vi "9174_9227_9205_CV_test.vi"() -> ()   [LabVIEW 2018]
uses:
  <vilib>/Utility/sysdir.llb/System Directory Type.ctl
panel:
  in  "觸發顯示訊號":bool=TRUE
  out "DW 2":bool
  out "ON":bool
  in  "自動存檔開關":bool=TRUE
  out "DW":bool
  in  "Stop":bool
  out "Time":timestamp format="%<%x %.3X>T"
  out "Real-Time":dynamicdata(graph)
  out "Real-Time":dynamicdata(graph)
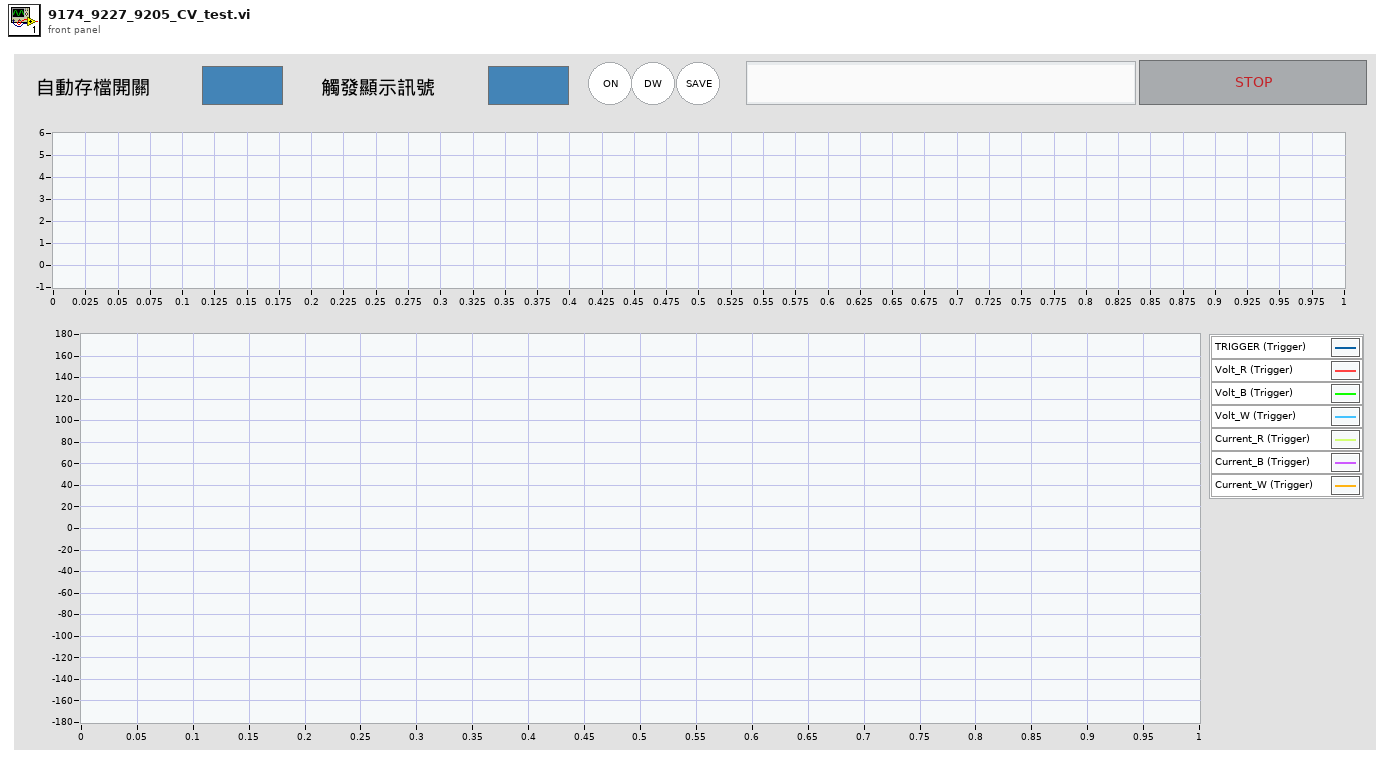
[diagram p1: front panel]
types:
  T1 = typedef "System Directory Type.ctl" = i32
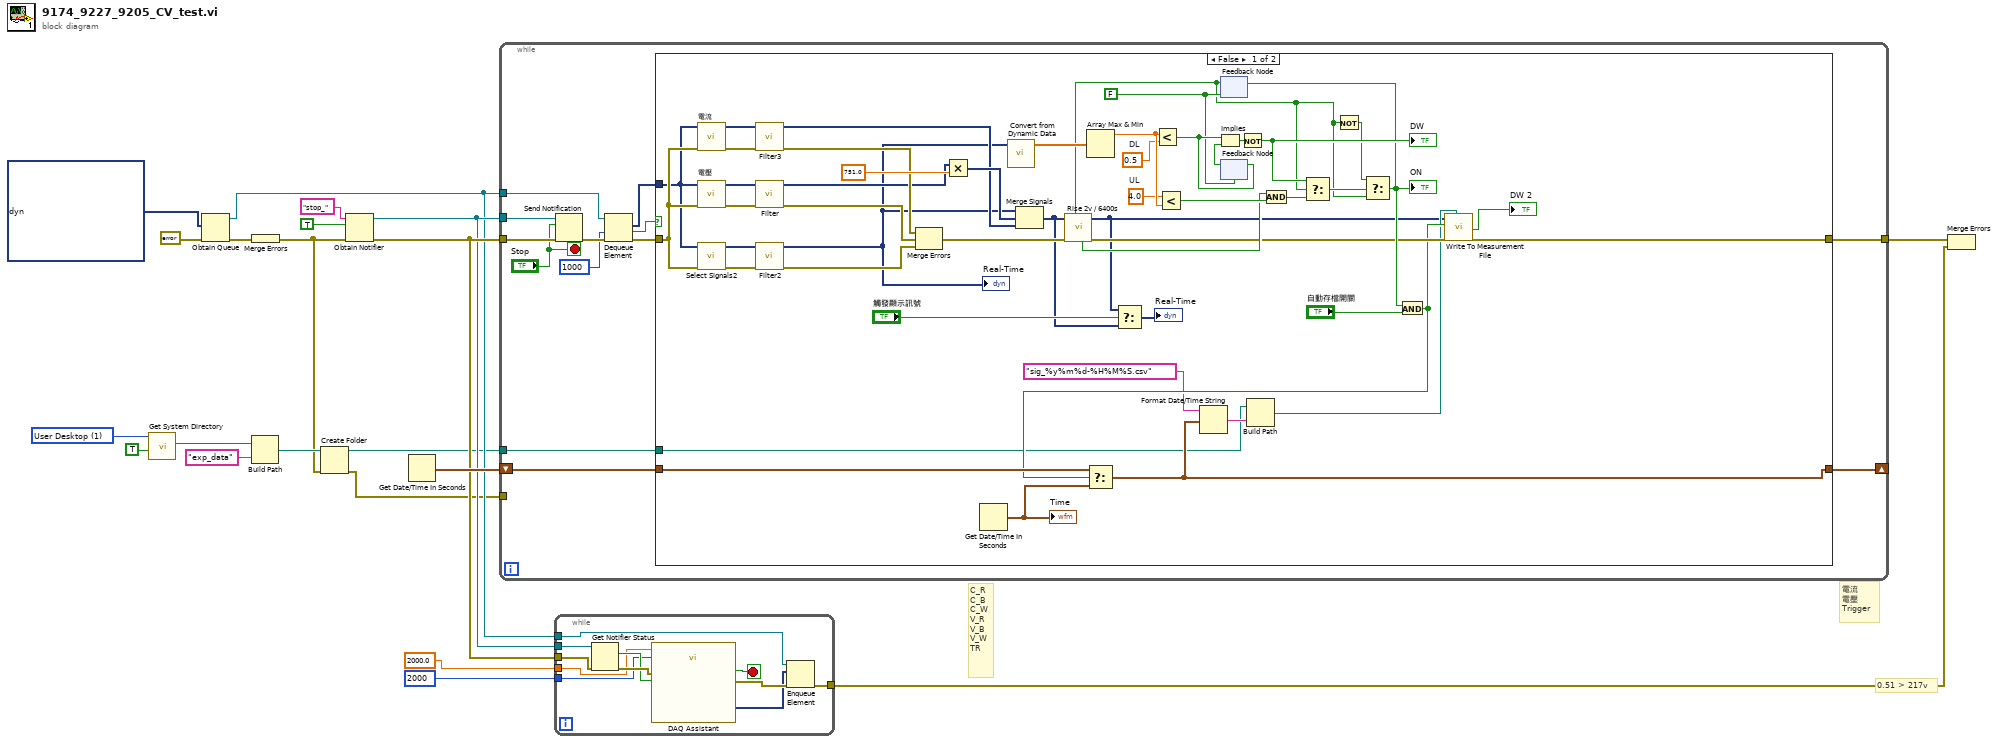
[diagram p0: block diagram]
diagram:
  w5 = T1 1 items=["User Home"=0, "User Desktop"=1, "User Documents"=2, "User Application Data"=3, "User Preferences"=4, "User Temporary"=5, "Public Documents"=6, "Public Application Data"=7, "Public Preferences"=8, "Public Cache"=13, "System Core Libraries"=9, "System Installed Libraries"=10, "Application Files"=11, "Boot Volume Root"=12] ("system directory type")
  # "C_R\nC_B\nC_W\nV_R\nV_B\nV_W\nTR"
  # "0.51 > 217v"
  # "電流\n電壓\nTrigger"
  n1 = call <vilib>:"Get System Directory.vi"("create directory if not found? (F)"=TRUE, "system directory type"=w5) -> ("system directory"=w7:path)  [unwired: 9 in]
  n2 = Obtain Queue(element data type=dynamicdata [] ("data"), error in (no error)=errorcluster {"status"=FALSE, "code"=0, "source"=""} ("Error In")) -> (queue out=w9:refnum<queue>, error out=w21:errorcluster)  [unwired: 3 in, 1 out]
  n3 = Build Path(base path=w7, name or relative path="exp_data") -> (appended path=w4:path)
  n4 = Merge Errors(w21) -> (w1:errorcluster)
  n5 = Create Folder(path (use dialog)=w4, error in=w1) -> (created path=w3:path, error out=w2:errorcluster)  [unwired: 1 in, 1 out]
  n6 = Obtain Notifier(name (unnamed)="stop_", notification data type=TRUE, error in (no error)=w1) -> (notifier out=w15:refnum<notifier>, error out=w16:errorcluster)  [unwired: 1 in, 1 out]
  n7 = Get Date/Time In Seconds() -> (seconds since 1Jan1904=w17:timestamp)
  n8 = while {
    tunnel: w16 -> [w34]
    tunnel: w15 -> [w33]
    tunnel: [w26] -> w10
    shift-right: [w31] -> _
    shift-left: w17 -> [w32]
    tunnel: w9 -> [w29]
    tunnel: w3 -> [w23]
    tunnel: w2 -> [_]
    stop <- "Stop" stop-if-true
    n9 = Send Notification(notification="Stop", notifier=w33, error in (no error)=w34) -> (error out=w30:errorcluster)  [unwired: 1 out]
    n10 = Dequeue Element(queue=w29, timeout in ms (-1)=1000, error in (no error)=w30) -> (element=w22:dynamicdata, timed out?=w27:bool, error out=w25:errorcluster)  [unwired: 1 out]
    n11 = case shown="False" w27 {
      tunnel: w32 -> [w83 w85]
      tunnel: [w42 w85] -> w31
      tunnel: w22 -> [w78 _]
      tunnel: [w68 w84] -> w26
      tunnel: w25 -> [w79 w84]
      tunnel: w23 -> [w40 _]
      frame False {
        w53 = FALSE
        w52 = 4.0  # UL
        w51 = 0.5  # DL
        n12 = call "電流"("error in (no error)"=w79, "Signals"=w78) -> ("error out"=w74:errorcluster, "Signal Out"=w76:dynamicdata)  [unwired: 8 in]
        n13 = call "電壓"("error in (no error)"=w79, "Signals"=w78) -> ("error out"=w80:errorcluster, "Signal Out"=w82:dynamicdata)  [unwired: 8 in]
        n14 = call "Select Signals2"("error in (no error)"=w79, "Signals"=w78) -> ("error out"=w77:errorcluster, "Signal Out"=w70:dynamicdata)  [unwired: 8 in]
        n15 = call "Filter3"("error in (no error)"=w74, "Signal"=w76) -> ("error out"=w72:errorcluster, "Filtered Signal"=w66:dynamicdata)  [unwired: 8 in]
        n16 = call "Filter"("error in (no error)"=w80, "Signal"=w82) -> ("error out"=w81:errorcluster, "Filtered Signal"=w69:dynamicdata)  [unwired: 8 in]
        n17 = call "Filter2"("error in (no error)"=w77, "Signal"=w70) -> ("error out"=w73:errorcluster, "Filtered Signal"=w49:dynamicdata)  [unwired: 8 in]
        "Real-Time" <- w49
        n18 = Merge Errors(w72, w81, w73) -> (w65:errorcluster)
        n19 = Multiply(x=w69, y=751.0) -> (x*y=w67:dynamicdata)
        n20 = Get Date/Time In Seconds() -> (seconds since 1Jan1904=w71:timestamp)
        "Time" <- w71
        n21 = call "Convert from Dynamic Data"("Dynamic Data Type"=w49) -> ("Array"=w59:dbl[])  [unwired: 3 in]
        n22 = Merge Signals(w49, w67, w66) -> (w36:dynamicdata)
        n23 = Array Max & Min(array=w59) -> (max value=w57:dbl)  [unwired: 3 out]
        n24 = Less?(x=w57, y=w51) -> (x < y?=w60:bool)
        n25 = Less?(x=w52, y=w57) -> (x < y?=w56:bool)
        n26 = feedback #1(w53) -> (w48:bool)
        n27 = call "Rise 2v / 6400s"("Manual Trigger"=w48, "error in (no error)"=w65, "Signals"=w36) -> ("error out"=w46:errorcluster, "Triggered Signals"=w37:dynamicdata, "Data Available"=w47:bool)  [unwired: 5 in, 1 out]
        n28 = Select(t=w37, s="觸發顯示訊號", f=w36) -> (s? t:f=→"Real-Time":dynamicdata)
        n29 = feedback #2(w53) -> (w61:bool)
        n30 = Implies(1:w61, 2:w60) -> (0:w62:bool)
        n31 = feedback-in #2(w60) -> ()
        n32 = Not(x=w62) -> (.not. x?=w64:bool)
        "DW" <- w64
        n33 = And(x=w47, y=w56) -> (x .and. y?=w55:bool)
        n34 = Select(t=w64, s=w48, f=w55) -> (s? t:f=w58:bool)
        n35 = Not(x=w48) -> (.not. x?=w54:bool)
        n36 = Select(t=w54, s=w58, f=w48) -> (s? t:f=w50:bool)
        "ON" <- w50
        n37 = feedback-in #1(w50) -> ()
        n38 = And(x=w50, y="自動存檔開關") -> (x .and. y?=w44:bool)
        n39 = Select(t=w83, s=w44, f=w71) -> (s? t:f=w42:timestamp)
        n40 = Format Date/Time String(time format string (%c)="sig_%y%m%d-%H%M%S.csv" ("string"), seconds (now)=w42) -> (date/time string=w43:string)  [unwired: 1 in]
        n41 = Build Path(base path=w40, name or relative path=w43) -> (appended path=w39:path)
        n42 = call "Write To Measurement File"("Signals"=w37, "Enable"=w44, "error in (no error)"=w46, "Filename"=w39) -> ("Saving Data"=→"DW 2":bool, "error out"=w68:errorcluster)  [unwired: 13 in, 1 out]
      }
      frame True {
      }
    }
  }
  n43 = while {
    tunnel: w9 -> [w95]
    tunnel: w16 -> [w92]
    tunnel: w15 -> [w91]
    tunnel: 2000 ("Sample to Read") -> [w89]
    tunnel: 2000.0 ("Sample Rate") -> [w88]
    tunnel: [w86] -> w11
    stop <- w96 stop-if-true
    n44 = Get Notifier Status(notifier=w91, error in (no error)=w92) -> (current notification=w90:bool, error out=w93:errorcluster)  [unwired: 3 out]
    n45 = call "DAQ Assistant"("rate"=w88, "number of samples"=w89, "error in"=w93, "stop (F)"=w90) -> ("data"=w87:dynamicdata, "stopped"=w96:bool, "error out"=w94:errorcluster)  [unwired: 12 in, 1 out]
    n46 = Enqueue Element(queue=w95, element=w87, error in (no error)=w94) -> (error out=w86:errorcluster)  [unwired: 1 in, 2 out]
  }
  n47 = Merge Errors(w10, w11) -> ()  [unwired: 1 out]
